vi "Configure Modulation (DSBAM).vi"(5 "Channel (1:Channel 1)":i32(ring)=1 items=["Channel 1"=1, "Channel 2"=2], 6 "Modulation Frequency (100 Hz)":dbl=100.0, 7 "Enable DSBAM Modulation (T:Enable)":bool=TRUE, 8 "error in (no error)":errorcluster, 9 "Modulation Waveform (0: Sine)":u16(ring) items=["Sine", "Square", "Triangle", "UpRamp", "DnRamp", "Noise", "Arb"], 10 "DSBAM Source (0: Internal)":u16(ring) items=["Internal", "External"], 11 "VISA resource name":refnum<visa-resource-name>) -> (0 "error out":errorcluster, 3 "VISA resource name out":refnum<visa-resource-name>)   [LabVIEW 2015, in "SDG X Series.lvlib"]
doc: "Configures and enables double side band amplitude modulation (DSBAM). In DSBAM, the amplitude of the carrier is varied by the amplitude of the modulating waveform. \n\n<B>Note:</B> The carrier waveform shape and parameters are set by the Configure Standard Waveform VI."
uses:
  <instrlib>/SDG X Series/SDG X Series.lvlib
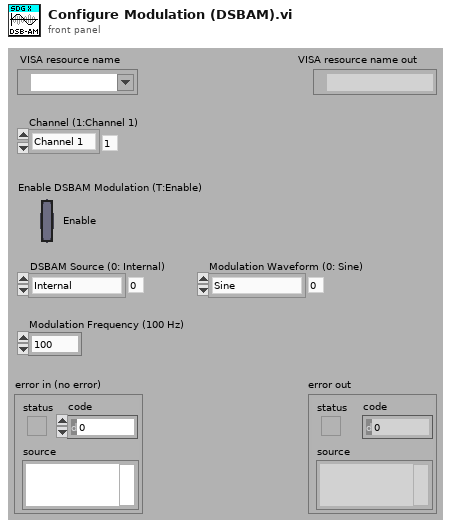
[diagram p1: front panel]
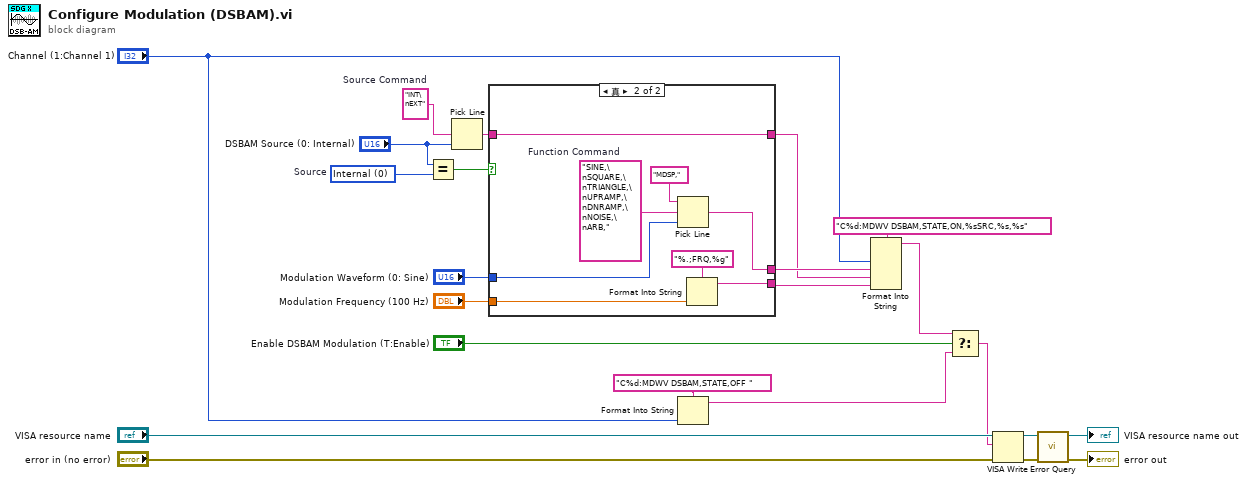
[diagram p0: block diagram]
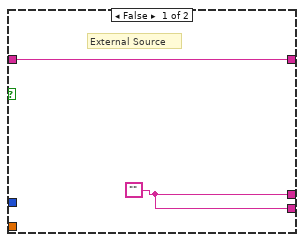
[diagram p2: hidden frame]
diagram:
  w12 = u16 0 items=["Internal", "External"]  # Source
  w13 = "INT\nEXT"  # Source Command
  n1 = Equal?(x="DSBAM Source (0: Internal)", y=w12) -> (x = y?=w11:bool)
  n2 = Pick Line(multi-line string=w13, line index="DSBAM Source (0: Internal)") -> (output string=w10:string)  [unwired: 1 in]
  n3 = case shown="真" w11 {
    tunnel: w10 -> [w25 w31]
    tunnel: "Modulation Waveform (0: Sine)" -> [_ w32]
    tunnel: "Modulation Frequency (100 Hz)" -> [_ w28]
    tunnel: [w25 w31] -> w7
    tunnel: [w24 w29] -> w8
    tunnel: [w24 w26] -> w6
    frame False {
      w24 = ""
      # "External Source"
    }
    frame True {
      w33 = "SINE,\nSQUARE,\nTRIANGLE,\nUPRAMP,\nDNRAMP,\nNOISE,\nARB,"  # Function Command
      n4 = Pick Line(string ("")="MDSP,", multi-line string=w33, line index=w32) -> (output string=w29:string)
      n5 = Format Into String(format string="%.;FRQ,%g", w28) -> (resulting string=w26:string)  [unwired: 2 in, 1 out]
    }
  }
  n6 = Format Into String(format string="C%d:MDWV DSBAM,STATE,OFF ", "Channel (1:Channel 1)") -> (resulting string=w4:string)  [unwired: 2 in, 1 out]
  n7 = Format Into String(format string="C%d:MDWV DSBAM,STATE,ON,%sSRC,%s,%s", "Channel (1:Channel 1)", w8, w7, w6) -> (resulting string=w3:string)  [unwired: 2 in, 1 out]
  n8 = Select(t=w3, s="Enable DSBAM Modulation (T:Enable)", f=w4) -> (s? t:f=w2:string)
  n9 = VISA Write(VISA resource name="VISA resource name", write buffer=w2, error in (no error)="error in (no error)") -> (VISA resource name out=w21:refnum<visa-resource-name>, error out=w20:errorcluster)  [unwired: 1 out]
  n10 = call <instrlib>:"Error Query.vi"("error in (no error)"=w20, "VISA resource name"=w21) -> ("error out"=→"error out":errorcluster, "VISA resource name out"=→"VISA resource name out":refnum<visa-resource-name>)  [unwired: 6 in, 2 out]
